vi "Variable list Modem Status analog.vi"() -> (6 "Variant":variant, 10 "Array":T1[](array[typedef]) {"Default Scaling"."Offset" format="%.5f"; "Default Scaling"."Gain" format="%.5f"})   [LabVIEW 2011]
uses:
  Measurments Handling/Fixed Analog Channel Definition.ctl
  Measurments Handling/Units/Quantity enum.ctl
  Measurments Handling/Update frequensies.ctl
  Measurments Handling/Channel catagory Enum.ctl
  Measurments Handling/Scaling.ctl
  Measurments Handling/Channel Classification Enum.ctl
  Variable List Modem Status Analog.ctl
  Measurments Handling/Common/Variable List Common Analog.ctl
  Tool/Variable List Tool Analog.ctl
  <vilib>/Utility/VariantDataType/GetNumericInfo.vi
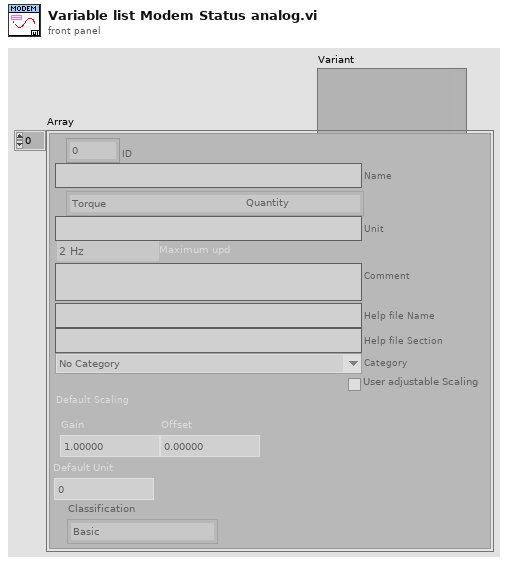
[diagram p1: front panel]
types:
  T1 = typedef "Fixed Analog Channel Definition.ctl" = cluster{"ID":u16, "Name":string, "Quantity":T2, "Unit":string, "Maximum upd":T3, "Comment":string, "Help file Name":string, "Help file Section ":string, "Category":T4, "User adjustable Scaling":bool, "Default Scaling":T5, "Default Unit":i32, "Classification":T6}
  T2 = typedef "Quantity enum.ctl" = enum16{"NA", "Acceleration", "Angle", "Current", "Force", "Distance", "Pressure", "Resistance", "Rotational Speed", "Speed", "Temperature", "Tension", "Torque", "Voltage", "Weight"}
  T3 = typedef "Update frequensies.ctl" = enum16{"2 Hz", "1 Hz", "0.1 Hz"}
  T4 = typedef "Channel catagory Enum.ctl" = enum16{"No Category", "Power", "Temperature", "Pressure"}
  T5 = typedef "Scaling.ctl" = cluster{"Gain":dbl, "Offset":dbl}
  T6 = typedef "Channel Classification Enum.ctl" = enum16{"Basic", "Advanced", "Expert", "Unused"}
  T7 = typedef "Variable List Tool Analog.ctl" = enum16{"Tool Max Temperature", "Tool (Controller) Temperature", "Tool Supply Voltage", "Tool (Controller) Current", "Tool Acceleration X", "Tool Acceleration Y", "Tool Acceleration Z", "Tool Acceleration Sum", "Tool Inclination", "Tool Rotation", "Tool GP Sensor 1", "Tool GP Sensor 2", "Tool (Pressure 1) Temperature", "Tool Pressure 1 RAW", "Tool (Pressure 2) Temperature", "Tool Pressure 2 RAW", "Tool (Solenoid) Temperature", "Tool Solenoid Position", "PSU Temp", "Head Voltage", "PSU Main Voltage out", "PSU Main Current out", "Upper Tension Sub Temp", "Tool Upper Tension Sub Raw", "Lower Tension Sub Temp", "Tool Lower Tension Sub Raw", "Tool Var27 - Reserved", "Tool Var28 - Reserved", "Tool Var29 - Reserved", "Tool Var30 - Reserved", "Stroke Extension", "Stroke In Force", "Stroke Out Force", "Stroke Force", "Stroker Pressure 1", "Stroker Pressure 2", "Stroker Upper Tension Sub", "Stroker Lower Tension Sub", "Stroker Var09 - Reserved", "Stroker Var10 - Reserved", "Tractor Upper Tension Sub", "Tractor Lower Tension Sub", "Tractor Var03 - Reserved", "Tractor Var04 - Reserved", "Tool Temperature sensor", "Tool Motor Voltage", "Tool Motor Current", "Tool Motor Torque", "Tool weight on bit", "Tool Motor RPM"}
  T8 = typedef "Variable List Common Analog.ctl" = enum16{"HVPSU Head Voltage", "HVPSU TS Voltage", "HVPSU Current", "PCP Cable Resistance", "Winch Depth", "Winch Line Speed", "Winch Wire Tension"}
  T9 = typedef "Variable List Modem Status Analog.ctl" = enum16{"TS_Signal_Quality", "TS_PCB_Temp", "TS_Gain", "DH_Signal_Quality", "DH_PCB_Temp", "DH_Gain", "Link_Status"}
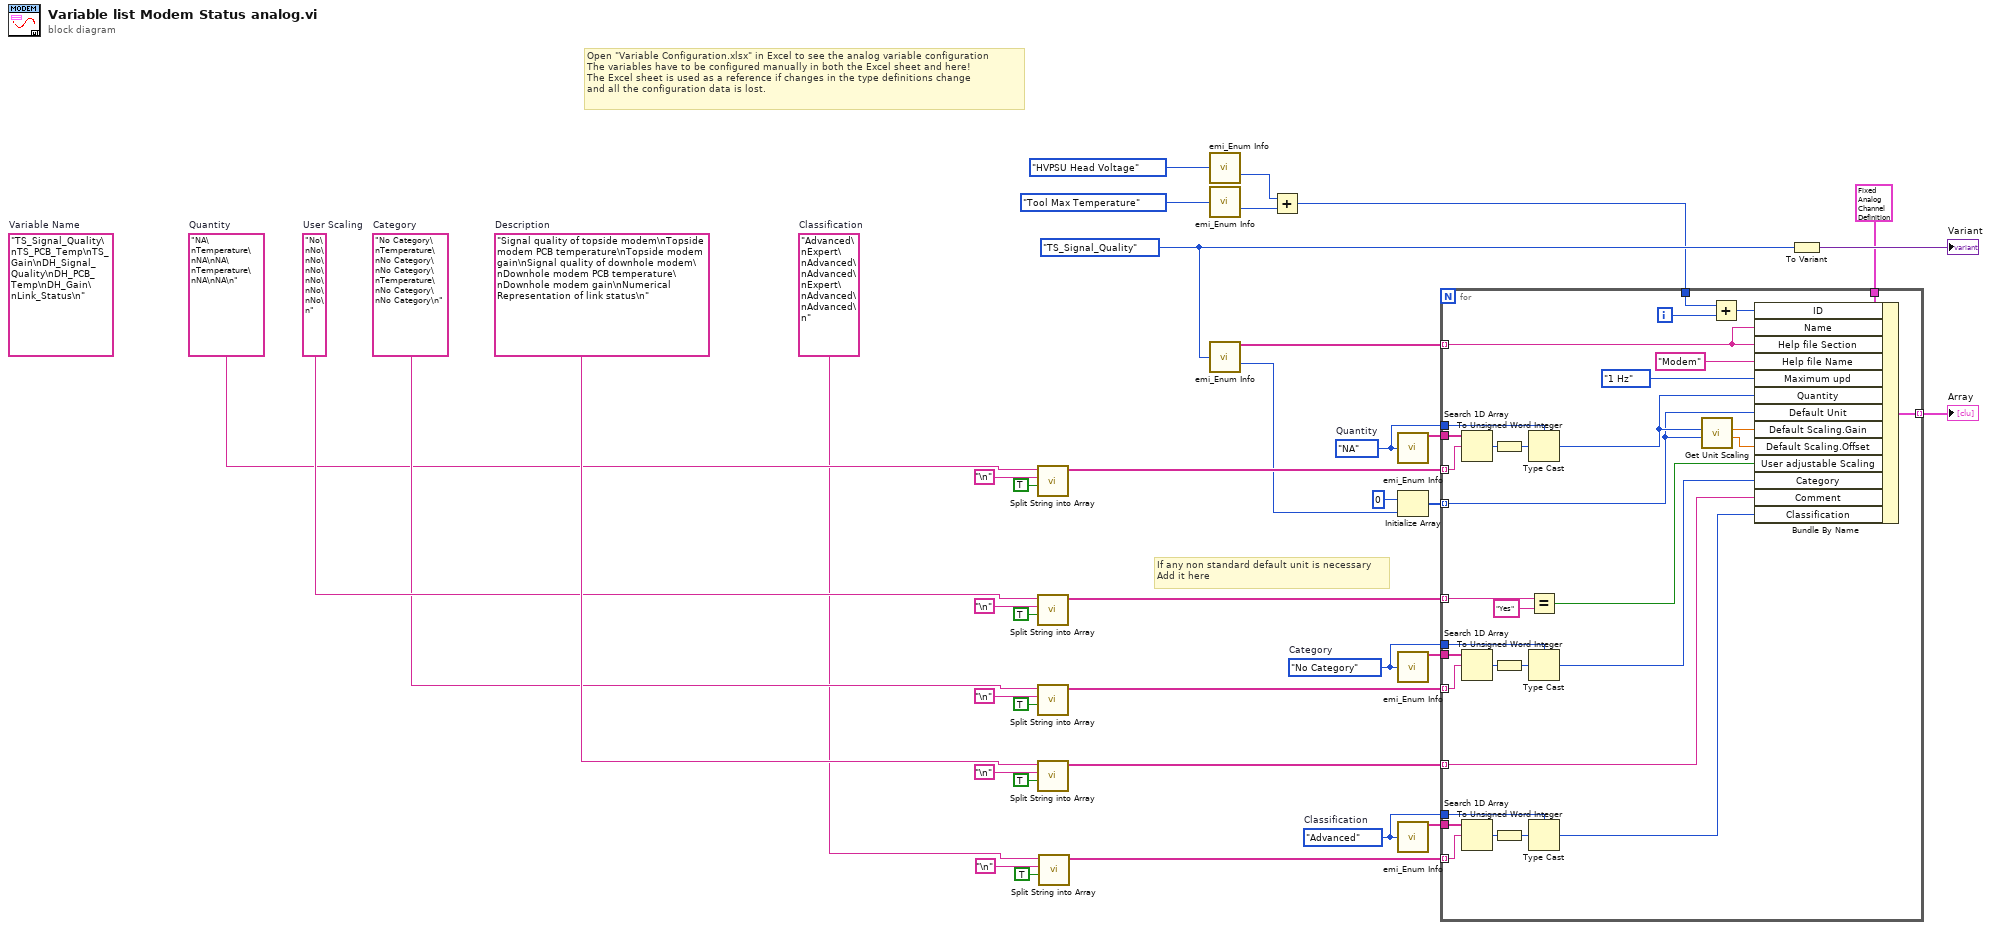
[diagram p0: block diagram]
diagram:
  w2 = Channel_Classification_Enum."Advanced"  # Classification
  w5 = "Advanced\nExpert\nAdvanced\nAdvanced\nExpert\nAdvanced\nAdvanced\n"  # Classification
  w17 = "No Category\nTemperature\nNo Category\nNo Category\nTemperature\nNo Category\nNo Category\n"  # Category
  w20 = Channel_catagory_Enum."No Category"  # Category
  w23 = "No\nNo\nNo\nNo\nNo\nNo\nNo\n"  # User Scaling
  w28 = Quantity_enum."NA"  # Quantity
  w15 = "NA\nTemperature\nNA\nNA\nTemperature\nNA\nNA\n"  # Quantity
  w27 = "Signal quality of topside modem\nTopside modem PCB temperature\nTopside modem gain\nSignal quality of downhole modem\nDownhole modem PCB temperature\nDownhole modem gain\nNumerical Representation of link status\n"  # Description
  (unwired) "TS_Signal_Quality\nTS_PCB_Temp\nTS_Gain\nDH_Signal_Quality\nDH_PCB_Temp\nDH_Gain\nLink_Status\n"  # Variable Name
  w36 = Variable_List_Modem_Status_Analog."TS_Signal_Quality" ("Variable ID")
  # "If any non standard default unit is necessary\nAdd it here"
  # "Open \"Variable Configuration.xlsx\" in Excel to see the analog variable configuration\nThe variables have to be configured manually in both the Excel sheet and here!\nThe Excel sheet is used as a reference if changes in the type definitions change\nand all the configuration data is lost."
  n1 = call "Split String into Array.vi"("Remove Last Row"=TRUE, "Separator"="\n", "Input string"=w15) -> ("Array of cells"=w30:string[])  [unwired: 8 in]
  n2 = call "Split String into Array.vi"("Remove Last Row"=TRUE, "Separator"="\n", "Input string"=w23) -> ("Array of cells"=w22:string[])  [unwired: 8 in]
  n3 = call "Split String into Array.vi"("Remove Last Row"=TRUE, "Separator"="\n", "Input string"=w17) -> ("Array of cells"=w16:string[])  [unwired: 8 in]
  n4 = call "Split String into Array.vi"("Remove Last Row"=TRUE, "Separator"="\n", "Input string"=w27) -> ("Array of cells"=w26:string[])  [unwired: 8 in]
  n5 = call "Split String into Array.vi"("Remove Last Row"=TRUE, "Separator"="\n", "Input string"=w5) -> ("Array of cells"=w3:string[])  [unwired: 8 in]
  n6 = call "emi_Enum Info.vi"("Enum"=Variable_List_Common_Analog."HVPSU Head Voltage" ("Action")) -> ("Numb Elements"=w10:i32)  [unwired: 11 in, 3 out]
  n7 = call "emi_Enum Info.vi"("Enum"=Variable_List_Tool_Analog."Tool Max Temperature" ("Variable ID")) -> ("Numb Elements"=w11:i32)  [unwired: 11 in, 3 out]
  n8 = call "emi_Enum Info.vi"("Enum"=w36) -> ("Text Elements"=w1:string[], "Numb Elements"=w8:i32)  [unwired: 11 in, 2 out]
  n9 = Add(x=w10, y=w11) -> (x+y=w9:i32)
  n10 = call "emi_Enum Info.vi"("Enum"=w28) -> ("Text Elements"=w29:string[])  [unwired: 11 in, 3 out]
  n11 = Initialize Array(0, w8) -> (w14:i32[])
  n12 = call "emi_Enum Info.vi"("Enum"=w20) -> ("Text Elements"=w21:string[])  [unwired: 11 in, 3 out]
  n13 = call "emi_Enum Info.vi"("Enum"=w2) -> ("Text Elements"=w4:string[])  [unwired: 11 in, 3 out]
  n14 = for {
    tunnel: [w72] -> w37 mode=indexing
    tunnel: T1 {"ID"=0, "Name"="", "Quantity"=enum."Acceleration", "Unit"="", "Maximum upd"=enum."2 Hz", "Comment"="", "Help file Name"="", "Help file Section "="", "Category"=enum."No Category", "User adjustable Scaling"=FALSE, "Default Scaling"={"Gain"=0.0, "Offset"=0.0}, "Default Unit"=0, "Classification"=enum."Basic"} ("Variable Defenition") -> [w71]
    tunnel: w26 -> [w54] mode=indexing
    tunnel: w14 -> [w61] mode=indexing
    tunnel: w30 -> [w68] mode=indexing
    tunnel: w29 -> [w69]
    tunnel: w28 -> [w66]
    tunnel: w22 -> [w60] mode=indexing
    tunnel: w16 -> [w56] mode=indexing
    tunnel: w21 -> [w55]
    tunnel: w20 -> [w57]
    tunnel: w9 -> [w49]
    tunnel: w3 -> [w44] mode=indexing
    tunnel: w4 -> [w45]
    tunnel: w2 -> [w43]
    tunnel: w1 -> [w41] mode=indexing
    i -> [w40]
    n15 = Search 1D Array(1D array=w69, element=w68) -> (index of element=w67:i32)  [unwired: 1 in]
    n16 = Search 1D Array(1D array=w55, element=w56) -> (index of element=w52:i32)  [unwired: 1 in]
    n17 = Search 1D Array(1D array=w45, element=w44) -> (index of element=w46:i32)  [unwired: 1 in]
    n18 = To Unsigned Word Integer(number=w67) -> (unsigned 16bit integer=w50:u16)
    n19 = To Unsigned Word Integer(number=w52) -> (unsigned 16bit integer=w51:u16)
    n20 = To Unsigned Word Integer(number=w46) -> (unsigned 16bit integer=w47:u16)
    n21 = Type Cast(type=w66, x=w50) -> (*(type *) &x=w64:T2)
    n22 = Equal?(x=w60, y="Yes") -> (x = y?=w58:bool)
    n23 = Type Cast(type=w57, x=w51) -> (*(type *) &x=w53:T4)
    n24 = Type Cast(type=w43, x=w47) -> (*(type *) &x=w42:T6)
    n25 = call "Get Unit Scaling.vi"("Unit Index"=w61, "Quantity"=w64) -> ("Offset"=w62:dbl, "Gain"=w63:dbl)  [unwired: 7 in, 1 out]
    n26 = Add(x=w49, y=w40) -> (x+y=w48:i32)
    n27 = Bundle By Name(cluster=w71, "ID"=w48, "Name"=w41, "Help file Section"=w41, "Help file Name"="Modem", "Maximum upd"=Update_frequensies."1 Hz", "Quantity"=w64, "Default Unit"=w61, "Default Scaling.Gain"=w63, "Default Scaling.Offset"=w62, "User adjustable Scaling"=w58, "Category"=w53, "Comment"=w54, "Classification"=w42) -> (w72:T1)
  }
  "Array" <- w37
  n28 = To Variant(anything=w36) -> (Variant=→"Variant":variant)
